vi "Read Item Tag.vi"(8 "error in (no error)":errorcluster, 11 "LabVIEWItem in":refnum<class "LabVIEWItem.lvclass">) -> (0 "error out":errorcluster, 2 "Item Tag":string, 3 "LabVIEWItem out":refnum<class "LabVIEWItem.lvclass">)   [LabVIEW 2020, in "Panther Dashboard.lvlib" / "LabVIEWItem.lvclass"]
uses:
  LabVIEWItem.lvclass
  LabVIEWItem.lvclass/LabVIEWItem.ctl
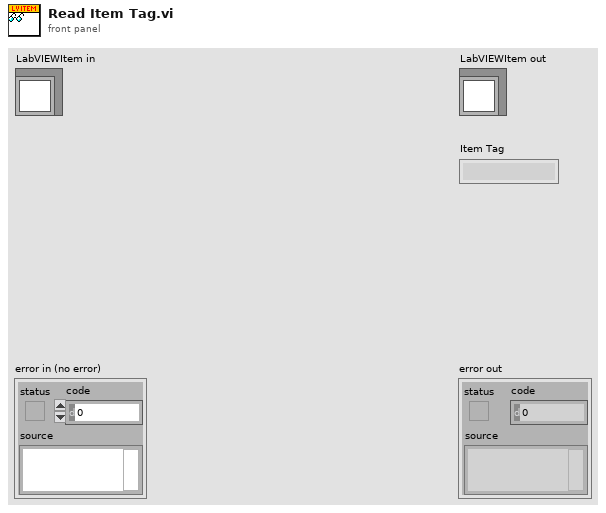
[diagram p1: front panel]
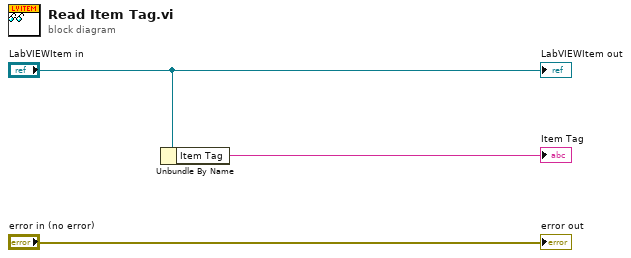
[diagram p0: block diagram]
diagram:
  n1 = Unbundle By Name("LabVIEWItem in") -> ("Item Tag"=→"Item Tag":string)
  "error out" <- "error in (no error)"
  "LabVIEWItem out" <- "LabVIEWItem in"
